vi "Scale.vi"() -> ()   [LabVIEW 2016, in "features.lvlib"]
doc: "This vi takes the current values from he beamline magnetic elements and converts them to a new value based on a specfic mass. It assumes a fixed terminal voltage"
uses:
  Features/features/features.lvlib
  controls/scale states.ctl
  <vilib>/Utility/miscctls.llb/LVRowAndColumnTypeDef.ctl
  Beam Line Sections/R45.vi
  Transmission/transmission.lvlib
  R30/R30  library.lvlib
  sub-VIs/sub-VIs.lvlib
  High energy end/High energy llb.lvlib
  controls/beamline sections.lvlib
panel:
  out "Un-Scale error":errorcluster
  out "Scaling Table":i32(listbox)
  out "Get values error":errorcluster
  out "Scaling error":errorcluster
  out "Scaled?":bool
  in  "Un-scale":bool
  out "Mass scaled to":dbl=1.0
  out "Mass scaled from":dbl=1.0
  in  "Desired Mass":dbl=1.0
  in  "Mass Currently on":dbl=1.0
  in  "Scale all":bool
  in  "stop":bool
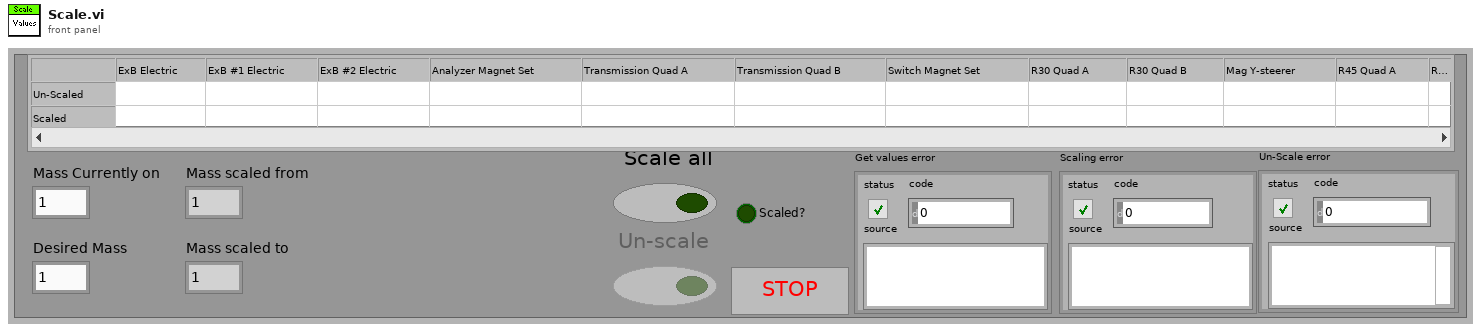
[diagram p1: front panel]
types:
  T1 = typedef "scale states.ctl" = enum16{"wait", "scale", "reset mass bkgd"}
  T2 = enum8{"Enabled", "Disabled", "Disabled and Grayed Out"}
  T3 = typedef "LVRowAndColumnTypeDef.ctl" = cluster{"Row":i32, "Column":i32}
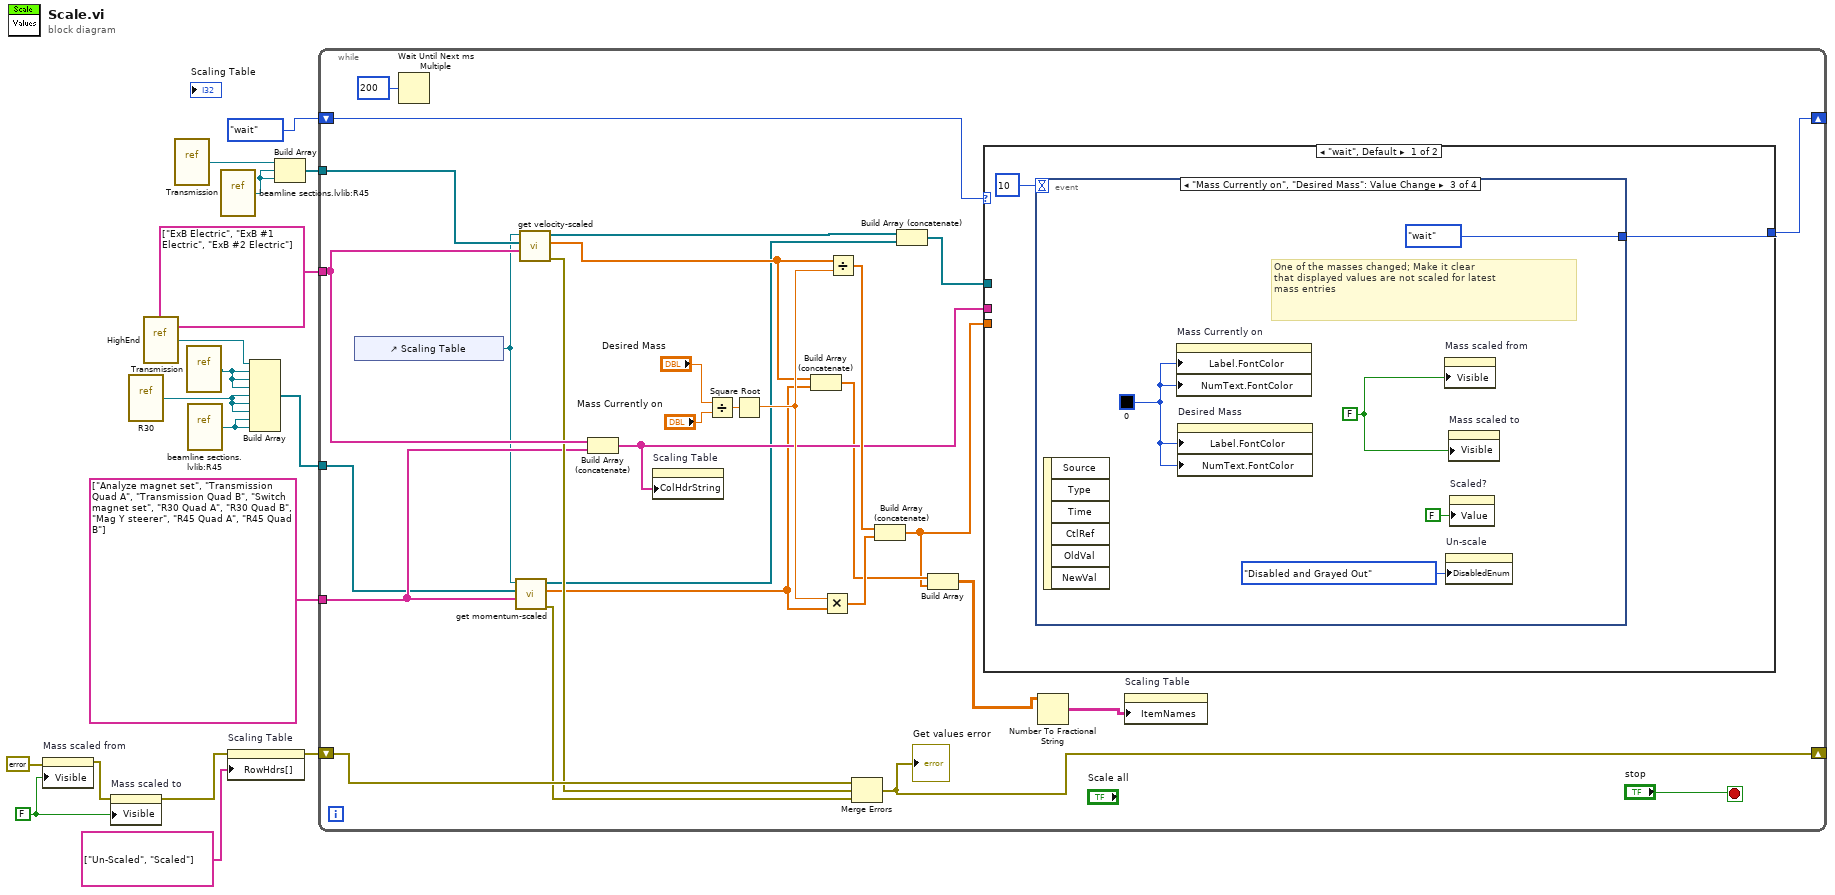
[diagram p0: block diagram]
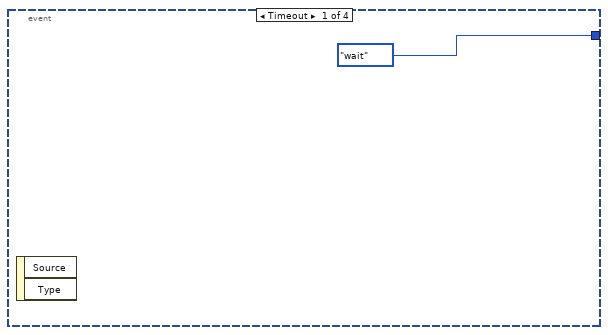
[diagram p2: hidden frame]
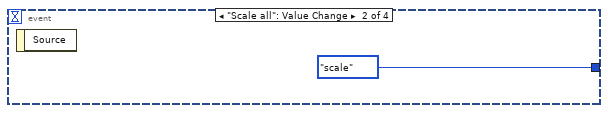
[diagram p3: hidden frame]
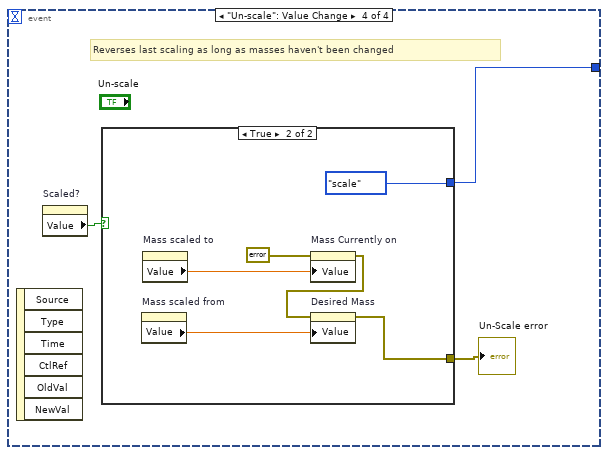
[diagram p4: hidden frame]
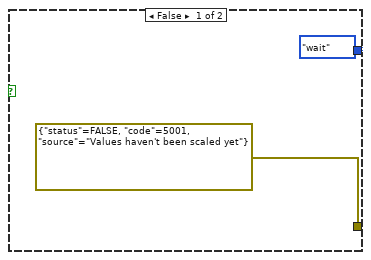
[diagram p5: hidden frame]
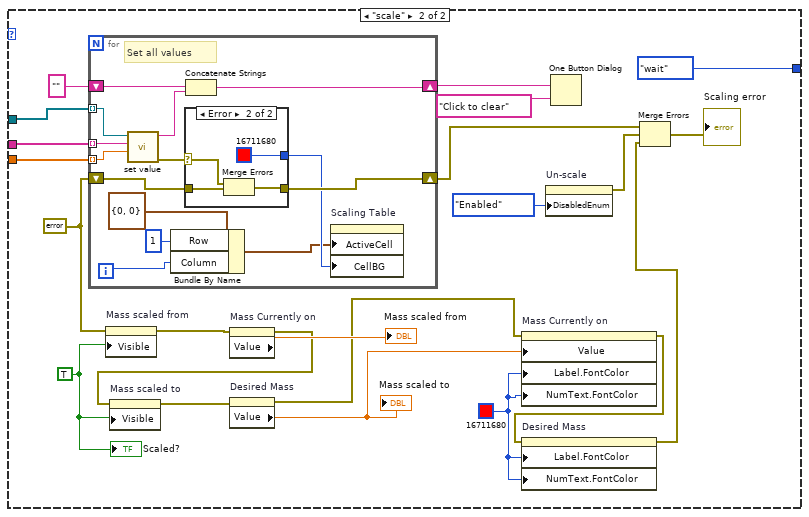
[diagram p6: hidden frame]
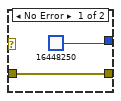
[diagram p7: hidden frame]
diagram:
  w4 = FALSE
  n1 = property on="Mass scaled from" class="DigNum (strict)"(error in=errorcluster {"status"=FALSE, "code"=0, "source"=""} ("error out"), "Visible"=w4) -> (error out=w7:errorcluster)  [unwired: 1 in, 1 out]
  n2 = property on="Mass scaled to" class="DigNum (strict)"(error in=w7, "Visible"=w4) -> (error out=w6:errorcluster)  [unwired: 1 in, 1 out]
  n3 = vi-ref "R30.vi"() -> (w1:refnum<vi>)
  n4 = vi-ref "HighEnd.vi"() -> (w11:refnum<vi>)
  n5 = vi-ref "Transmission.vi"() -> (w14:refnum<vi>)
  n6 = vi-ref "Transmission.vi"() -> (w12:refnum<vi>)
  n7 = vi-ref "beamline sections.lvlib:R45.vi"() -> (w2:refnum<vi>)
  n8 = vi-ref "beamline sections.lvlib:R45.vi"() -> (w15:refnum<vi>)
  n9 = property on="Scaling Table" class="MCListbox (strict)"(error in=w6, "RowHdrs[]"=string[] ["Un-Scaled", "Scaled"]) -> (error out=w9:errorcluster)  [unwired: 1 in, 1 out]
  n10 = Build Array(w11, w12, w12, w12, w1, w1, w1, w2, w2) -> (w10:refnum<vi>[])
  n11 = Build Array(w14, w15, w15) -> (w13:refnum<vi>[])
  n12 = while {
    shift-right: [w36] -> _
    shift-left: w9 -> [w37]
    tunnel: string[] ["Analyze magnet set", "Transmission Quad A", "Transmission Quad B", "Switch magnet set", "R30 Quad A", "R30 Quad B", "Mag Y steerer", "R45 Quad A", "R45 Quad B"] -> [w23]
    tunnel: string[] ["ExB Electric", "ExB #1 Electric", "ExB #2 Electric"] -> [w27]
    tunnel: w13 -> [w28]
    tunnel: w10 -> [w22]
    shift-right: [w31] -> _
    shift-left: scale_states."wait" -> [w32]
    stop <- "stop" stop-if-true
    n13 = control-ref of="Scaling Table"() -> (w18:refnum<vi>)
    n14 = Wait Until Next ms Multiple(millisecond multiple=u32 200) -> ()  [unwired: 1 out]
    n15 = call "get momentum-scaled.vi"("Array 2"=w23, "Array"=w22, "MulticolumnListbox in"=w18) -> ("error out"=w21:errorcluster, "Array 3"=w20:ext[], "Array 4"=w19:refnum<vi>[])  [unwired: 6 in]
    n16 = call "get velocity-scaled.vi"("Array"=w27, "Array 2"=w28, "MulticolumnListbox in"=w18) -> ("error out"=w26:errorcluster, "Array 3"=w24:ext[], "Array 4"=w25:refnum<vi>[])  [unwired: 6 in]
    n17 = Build Array (concatenate)(w27, w23) -> (w38:string[])
    n18 = property on="Scaling Table" class="MCListbox (strict)"("ColHdrString"=w38) -> ()  [unwired: 2 in, 2 out]
    n19 = Divide(x="Desired Mass", y="Mass Currently on") -> (x/y=w44:dbl)
    n20 = Square Root(x=w44) -> (sqrt(x)=w43:dbl)
    n21 = Build Array (concatenate)(w24, w20) -> (w35:ext[])
    n22 = Multiply(x=w43, y=w20) -> (x*y=w41:ext[])
    n23 = Divide(x=w24, y=w43) -> (x/y=w42:ext[])
    n24 = Merge Errors(w37, w26, w21) -> (w36:errorcluster)
    "Get values error" <- w36
    n25 = Build Array (concatenate)(w42, w41) -> (w34:ext[])
    n26 = Build Array (concatenate)(w25, w19) -> (w40:refnum<vi>[])
    n27 = Build Array(w35, w34) -> (w29:ext[][])
    n28 = case shown="\"wait\", Default" w32 {
      tunnel: w40 -> [_ w72]
      tunnel: w38 -> [_ w71]
      tunnel: w34 -> [_ w70]
      tunnel: [w47 scale_states."wait"] -> w31
      frame "wait", Default {
        n29 = event shown="[2] \"Mass Currently on\", \"Desired Mass\": Value Change" {
          selector: _ -> [_ _ _ _]
          dyn-events: _ -> [_ _ _ _]
          timeout: 10 -> [_ _ _ _]
          tunnel: [scale_states."wait" scale_states."scale" scale_states."wait" w56] -> w47
          event Timeout {
            n30 = event-data() -> ()  [unwired: 1 in, 2 out]
          }
          event "Scale all": Value Change {
            n31 = event-data() -> ()  [unwired: 1 in, 1 out]
          }
          event "Mass Currently on", "Desired Mass": Value Change {
            w52 = u32 0
            w55 = FALSE
            # "One of the masses changed; Make it clear \nthat displayed values are not scaled for latest\nmass entries"
            n32 = event-data() -> ()  [unwired: 1 in, 6 out]
            n33 = property on="Mass Currently on" class="DigNum (strict)"("Label.FontColor"=w52, "NumText.FontColor"=w52) -> ()  [unwired: 2 in, 2 out]
            n34 = property on="Desired Mass" class="DigNum (strict)"("Label.FontColor"=w52, "NumText.FontColor"=w52) -> ()  [unwired: 2 in, 2 out]
            n35 = property on="Mass scaled from" class="DigNum (strict)"("Visible"=w55) -> ()  [unwired: 2 in, 2 out]
            n36 = property on="Un-scale" class="Bool"("DisabledEnum"=T2."Disabled and Grayed Out" ("Disabled")) -> ()  [unwired: 2 in, 2 out]
            n37 = property on="Mass scaled to" class="DigNum (strict)"("Visible"=w55) -> ()  [unwired: 2 in, 2 out]
            n38 = property on="Scaled?" class="Bool (strict)"("Value"=FALSE ("Scaled?")) -> ()  [unwired: 2 in, 2 out]
          }
          event "Un-scale": Value Change {
            # "Reverses last scaling as long as masses haven't been changed"
            n39 = event-data() -> ()  [unwired: 1 in, 6 out]
            n40 = property on="Scaled?" class="Bool (strict)"() -> ("Value"=w58:bool)  [unwired: 2 in, 2 out]
            n41 = case shown="True" w58 {
              tunnel: [errorcluster {"status"=FALSE, "code"=5001, "source"="Values haven't been scaled yet"} ("error out") w61] -> w57
              tunnel: [scale_states."wait" scale_states."scale"] -> w56
              frame False {
              }
              frame True {
                n42 = property on="Mass scaled from" class="DigNum (strict)"() -> ("Value"=w66:dbl)  [unwired: 2 in, 2 out]
                n43 = property on="Mass scaled to" class="DigNum (strict)"() -> ("Value"=w65:dbl)  [unwired: 2 in, 2 out]
                n44 = property on="Mass Currently on" class="DigNum (strict)"(error in=errorcluster {"status"=FALSE, "code"=0, "source"=""} ("error out"), "Value"=w65) -> (error out=w64:errorcluster)  [unwired: 1 in, 1 out]
                n45 = property on="Desired Mass" class="DigNum (strict)"(error in=w64, "Value"=w66) -> (error out=w61:errorcluster)  [unwired: 1 in, 1 out]
              }
            }
            "Un-Scale error" <- w57
          }
        }
      }
      frame "scale" {
        w77 = errorcluster {"status"=FALSE, "code"=0, "source"=""} ("error out")
        w73 = u32 16711680
        w83 = TRUE
        n46 = for {
          tunnel: w70 -> [w101] mode=indexing
          tunnel: w72 -> [w102] mode=indexing
          tunnel: w71 -> [w100] mode=indexing
          shift-right: [w97] -> w78
          shift-left: w77 -> [w98]
          shift-right: [w94] -> w68
          shift-left: "" -> [w96]
          i -> [w90]
          # "Set all values"
          n47 = call "set value.vi"("Set value"=w101, "Control Name"=w100, "VI Refnum"=w102) -> ("error out"=w99:errorcluster, "Output string"=w95:string)  [unwired: 7 in]
          n48 = Bundle By Name(cluster=T3 {"Row"=0, "Column"=0} ("Active Cell:Active Cell"), "Row"=1, "Column"=w90) -> (w91:T3)
          n49 = case shown="Error" w99 {
            selector: w99 -> [_ w106]
            tunnel: w98 -> [w104 w107]
            tunnel: [w104 w108] -> w97
            tunnel: [u32 16448250 u32 16711680] -> w93
            frame No Error {
            }
            frame Error {
              n50 = Merge Errors(w106, w107) -> (w108:errorcluster)
            }
          }
          n51 = Concatenate Strings(w96, w95) -> (w94:string)
          n52 = property on="Scaling Table" class="MCListbox (strict)"("ActiveCell"=w91, "CellBG"=w93) -> ()  [unwired: 2 in, 2 out]
        }
        n53 = property on="Mass scaled from" class="DigNum (strict)"(error in=w77, "Visible"=w83) -> (error out=w86:errorcluster)  [unwired: 1 in, 1 out]
        n54 = property on="Mass Currently on" class="DigNum (strict)"(error in=w86) -> (error out=w82:errorcluster, "Value"=→"Mass scaled from":dbl)  [unwired: 1 in, 1 out]
        n55 = property on="Mass scaled to" class="DigNum (strict)"(error in=w82, "Visible"=w83) -> (error out=w85:errorcluster)  [unwired: 1 in, 1 out]
        n56 = property on="Desired Mass" class="DigNum (strict)"(error in=w85) -> (error out=w81:errorcluster, "Value"=w84:dbl)  [unwired: 1 in, 1 out]
        "Mass scaled to" <- w84
        n57 = property on="Mass Currently on" class="DigNum (strict)"(error in=w81, "Value"=w84, "Label.FontColor"=w73, "NumText.FontColor"=w73) -> (error out=w80:errorcluster)  [unwired: 1 in, 1 out]
        n58 = property on="Desired Mass" class="DigNum (strict)"(error in=w80, "Label.FontColor"=w73, "NumText.FontColor"=w73) -> (error out=w74:errorcluster)  [unwired: 1 in, 1 out]
        n59 = property on="Un-scale" class="Bool"("DisabledEnum"=T2."Enabled" ("Disabled")) -> (error out=w75:errorcluster)  [unwired: 2 in, 1 out]
        n60 = One Button Dialog(message=w68, button name ("OK")="Click to clear") -> ()  [unwired: 1 out]
        n61 = Merge Errors(w78, w75, w74) -> (→"Scaling error":errorcluster)
        "Scaled?" <- w83
      }
    }
    n62 = Number To Fractional String(number=w29) -> (F-format string=w30:string[][])  [unwired: 3 in]
    n63 = property on="Scaling Table" class="MCListbox (strict)"("ItemNames"=w30) -> ()  [unwired: 2 in, 2 out]
  }
